vi "Test I8 Value.vi"(7 "Name":string="Test I8 Value", 8 "Upper Limit":refnum<class "Abs_I8 Integer.lvclass">, 9 "Lower Limit":refnum<class "Abs_I8 Integer.lvclass">, 10 "Limit Test Type":T1, 11 "Tested Value":refnum<class "Abs_I8 Integer.lvclass">) -> (3 "abs_Node":refnum<class "abs_Node.lvclass">)   [LabVIEW 2021, in "BT.lvlib"]
uses:
  BT.lvlib
  Support/Nodes/abs_Node/abs_Node.lvclass
  Support/Limit Test Type.ctl
  <vilib>/TSA/Abstract Data Classes/Abs_Types/I8 Integer/Abs_I8 Integer.lvclass
  C:/Program Files (x86)/National Instruments/LabVIEW 2021/vi.lib/TSA/Abstract Data Classes/Abs_Types/Numeric/Abs_Numeric.lvclass
  Support/Nodes/Leaves/Test Boolean/Test Boolean.lvclass
  C:/Program Files (x86)/National Instruments/LabVIEW 2021/vi.lib/TSA/Abstract Data Classes/Abs_Types/Type/Abs_Type.lvclass
  C:/Users/Tim/Documents/GitHub/LV_Behaviour_Tree/Source/Support/abs_Type Leaf/abs_Type Leaf.lvclass
  C:/Users/Tim/Documents/GitHub/LV_Behaviour_Tree/Source/Support/abs_Node/abs_Node.lvclass
  <vilib>/TSA/Abstract Data Classes/Abs_Types/Type/Abs_Type.lvclass/Abs_Type.ctl
  Support/Nodes/Leaves/abs_Type Leaf/abs_Type Leaf.lvclass/abs_Type Leaf.ctl
  <vilib>/TSA/Abstract Data Classes/Abs_Types/Type/Properties/Write Name.vi
  Support/Nodes/Leaves/abs_Type Leaf/Properties/Write Value Class.vi
  <vilib>/TSA/Abstract Data Classes/Abs_Types/Boolean/Abs_Boolean.lvclass
  <vilib>/TSA/Abstract Data Classes/Functions/Compare/Support/Equal/I8/Method.vi
  <vilib>/TSA/Abstract Data Classes/Functions/Compare/Support/Not Equal/I8/Method.vi
  <vilib>/TSA/Abstract Data Classes/Functions/Compare/Support/Greater/I8/Method.vi
  <vilib>/TSA/Abstract Data Classes/Functions/Compare/Support/Less/I8/Method.vi
  <vilib>/TSA/Abstract Data Classes/Functions/Compare/Support/Greater Equal/I8/Method.vi
  <vilib>/TSA/Abstract Data Classes/Functions/Compare/Support/Less Equal/I8/Method.vi
  <vilib>/TSA/Abstract Data Classes/Functions/Logic/Support/AND/Bool/Method.vi
  <vilib>/TSA/Abstract Data Classes/Functions/Logic/Support/OR/Bool/Method.vi
  <vilib>/TSA/Abstract Data Classes/Functions/Math/Support/Add/I8/Method.vi
  <vilib>/TSA/Abstract Data Classes/Functions/Math/Support/Subtract/I8/Method.vi
  <vilib>/TSA/Abstract Data Classes/Functions/Logic/Support/AND/Bool/AND_Bool.lvclass
  <vilib>/TSA/Abstract Data Classes/Functions/Logic/Support/OR/Bool/OR_Bool.lvclass
  <vilib>/TSA/Abstract Data Classes/Functions/Compare/Support/Equal/I8/Equal_I8.lvclass
  <vilib>/TSA/Abstract Data Classes/Functions/Compare/Support/Not Equal/I8/Not Equal_I8.lvclass
  <vilib>/TSA/Abstract Data Classes/Functions/Compare/Support/Greater/I8/Greater_I8.lvclass
  <vilib>/TSA/Abstract Data Classes/Functions/Compare/Support/Less/I8/Less_I8.lvclass
  <vilib>/TSA/Abstract Data Classes/Functions/Compare/Support/Greater Equal/I8/Greater Equal_I8.lvclass
  <vilib>/TSA/Abstract Data Classes/Functions/Compare/Support/Less Equal/I8/Less Equal_I8.lvclass
  C:/Program Files (x86)/National Instruments/LabVIEW 2021/vi.lib/TSA/Abstract Data Classes/Abs_Types/Integer/Abs_Integer.lvclass
  C:/Program Files (x86)/National Instruments/LabVIEW 2021/vi.lib/TSA/Abstract Data Classes/Abs_Types/Value/Abs_Value.lvclass
  C:/Program Files (x86)/National Instruments/LabVIEW 2021/vi.lib/TSA/Abstract Data Classes/Abs_Types/I8 Integer/Abs_I8 Integer.lvclass
  <vilib>/TSA/Abstract Data Classes/Functions/Math/Support/Add/I8/Add_I8.lvclass
  <vilib>/TSA/Abstract Data Classes/Functions/Math/Support/Subtract/I8/Subtract_I8.lvclass
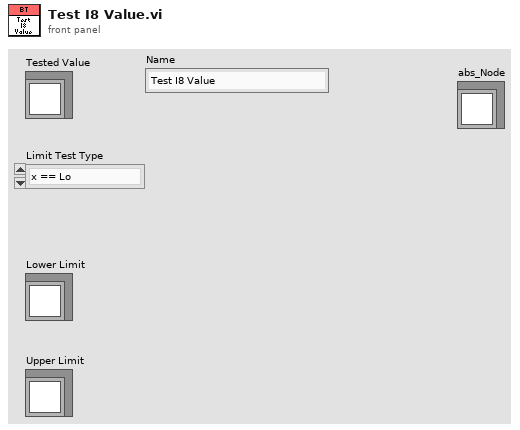
[diagram p1: front panel]
types:
  T1 = typedef "BT.lvlib/Limit Test Type.ctl" = enum16{"x == Lo", "x != Lo", "x > Lo", "x < Lo", "x >= Lo", "x <= Lo", "Lo > x < Hi", "Lo >= x <= Hi", "Lo >= x < Hi", "Lo > x <= Hi", "Lo < x > Hi", "Lo <= x >= Hi", "Lo <= x > Hi", "Lo < x >= Hi", "x == Lo +/- Hi"}
  T2 = typedef "Add_I8.lvclass/Abs_Type.ctl" = refnum<class "Abs_I8 Integer.lvclass">
  T3 = typedef "Subtract_I8.lvclass/Abs Type.ctl" = refnum<class "Abs_I8 Integer.lvclass">
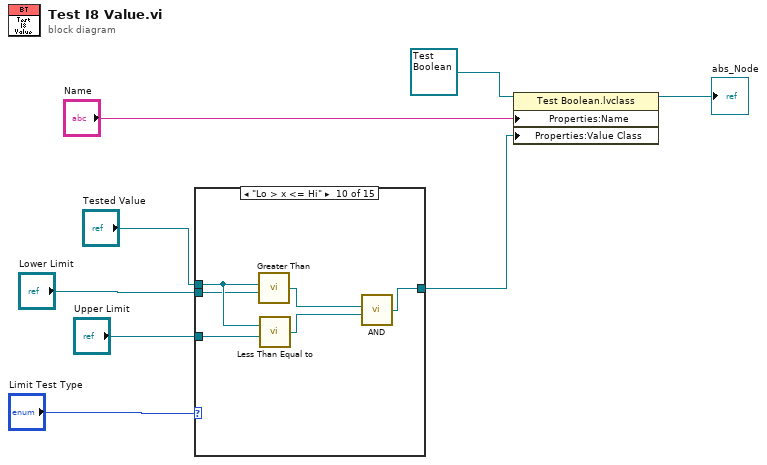
[diagram p0: block diagram]
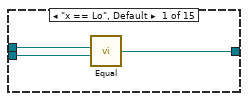
[diagram p2: hidden frame]
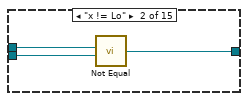
[diagram p3: hidden frame]
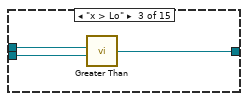
[diagram p4: hidden frame]
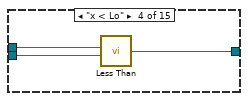
[diagram p5: hidden frame]
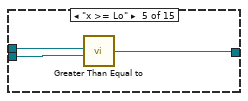
[diagram p6: hidden frame]
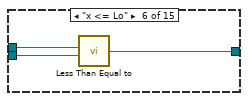
[diagram p7: hidden frame]
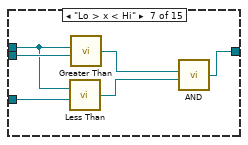
[diagram p8: hidden frame]
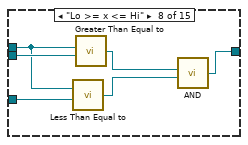
[diagram p9: hidden frame]
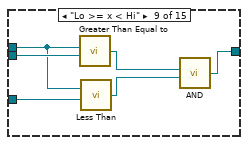
[diagram p10: hidden frame]
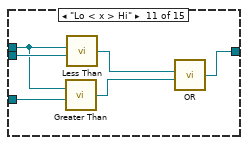
[diagram p11: hidden frame]
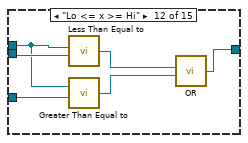
[diagram p12: hidden frame]
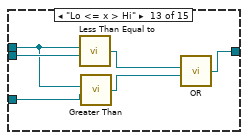
[diagram p13: hidden frame]
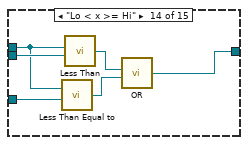
[diagram p14: hidden frame]
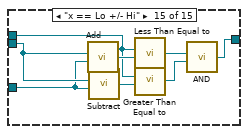
[diagram p15: hidden frame]
diagram:
  n1 = case shown="\"Lo > x <= Hi\"" "Limit Test Type" {
    tunnel: "Tested Value" -> [w11 w13 w17 w20 w23 w26 w31 w37 w43 w49 w53 w61 w66 w72 w79]
    tunnel: "Lower Limit" -> [w10 w14 w16 w19 w22 w25 w32 w38 w44 w48 w55 w62 w68 w73 w82]
    tunnel: [w9 w12 w15 w18 w21 w24 w27 w33 w39 w45 w56 w57 w63 w69 w75] -> w3
    tunnel: "Upper Limit" -> [_ _ _ _ _ _ w30 w36 w42 w50 w54 w60 w67 w74 w81]
    frame "x == Lo", Default {
      n2 = call-poly <vilib>:"Equal.vi"("Value B"=w10, "Value A"=w11) -> ("Result"=w9:refnum<class "Abs_Boolean.lvclass">)  [unwired: 4 in]
    }
    frame "x != Lo" {
      n3 = call-poly <vilib>:"Not Equal.vi"("Value B"=w14, "Value A"=w13) -> ("Result"=w12:refnum<class "Abs_Boolean.lvclass">)  [unwired: 4 in]
    }
    frame "x > Lo" {
      n4 = call-poly <vilib>:"Greater Than.vi"("Value B"=w16, "Value A"=w17) -> ("Result"=w15:refnum<class "Abs_Boolean.lvclass">)  [unwired: 4 in]
    }
    frame "x < Lo" {
      n5 = call-poly <vilib>:"Less Than.vi"("Value B"=w19, "Value A"=w20) -> ("Result"=w18:refnum<class "Abs_Boolean.lvclass">)  [unwired: 4 in]
    }
    frame "x >= Lo" {
      n6 = call-poly <vilib>:"Greater Than Equal to.vi"("Value B"=w22, "Value A"=w23) -> ("Result"=w21:refnum<class "Abs_Boolean.lvclass">)  [unwired: 4 in]
    }
    frame "x <= Lo" {
      n7 = call-poly <vilib>:"Less Than Equal to.vi"("Value B"=w25, "Value A"=w26) -> ("Result"=w24:refnum<class "Abs_Boolean.lvclass">)  [unwired: 4 in]
    }
    frame "Lo > x < Hi" {
      n8 = call-poly <vilib>:"Less Than.vi"("Value B"=w30, "Value A"=w31) -> ("Result"=w28:refnum<class "Abs_Boolean.lvclass">)  [unwired: 4 in]
      n9 = call-poly <vilib>:"Greater Than.vi"("Value B"=w32, "Value A"=w31) -> ("Result"=w29:refnum<class "Abs_Boolean.lvclass">)  [unwired: 4 in]
      n10 = call-poly <vilib>:"AND.vi"("B"=w28, "A"=w29) -> ("Result"=w27:refnum<class "Abs_Boolean.lvclass">)  [unwired: 4 in]
    }
    frame "Lo >= x <= Hi" {
      n11 = call-poly <vilib>:"Less Than Equal to.vi"("Value B"=w36, "Value A"=w37) -> ("Result"=w34:refnum<class "Abs_Boolean.lvclass">)  [unwired: 4 in]
      n12 = call-poly <vilib>:"Greater Than Equal to.vi"("Value B"=w38, "Value A"=w37) -> ("Result"=w35:refnum<class "Abs_Boolean.lvclass">)  [unwired: 4 in]
      n13 = call-poly <vilib>:"AND.vi"("B"=w34, "A"=w35) -> ("Result"=w33:refnum<class "Abs_Boolean.lvclass">)  [unwired: 4 in]
    }
    frame "Lo >= x < Hi" {
      n14 = call-poly <vilib>:"Greater Than Equal to.vi"("Value B"=w44, "Value A"=w43) -> ("Result"=w40:refnum<class "Abs_Boolean.lvclass">)  [unwired: 4 in]
      n15 = call-poly <vilib>:"Less Than.vi"("Value B"=w42, "Value A"=w43) -> ("Result"=w41:refnum<class "Abs_Boolean.lvclass">)  [unwired: 4 in]
      n16 = call-poly <vilib>:"AND.vi"("B"=w41, "A"=w40) -> ("Result"=w39:refnum<class "Abs_Boolean.lvclass">)  [unwired: 4 in]
    }
    frame "Lo > x <= Hi" {
      n17 = call-poly <vilib>:"Greater Than.vi"("Value B"=w48, "Value A"=w49) -> ("Result"=w47:refnum<class "Abs_Boolean.lvclass">)  [unwired: 4 in]
      n18 = call-poly <vilib>:"Less Than Equal to.vi"("Value B"=w50, "Value A"=w49) -> ("Result"=w46:refnum<class "Abs_Boolean.lvclass">)  [unwired: 4 in]
      n19 = call-poly <vilib>:"AND.vi"("B"=w46, "A"=w47) -> ("Result"=w45:refnum<class "Abs_Boolean.lvclass">)  [unwired: 4 in]
    }
    frame "Lo < x > Hi" {
      n20 = call-poly <vilib>:"Greater Than.vi"("Value B"=w54, "Value A"=w53) -> ("Result"=w51:refnum<class "Abs_Boolean.lvclass">)  [unwired: 4 in]
      n21 = call-poly <vilib>:"Less Than.vi"("Value B"=w55, "Value A"=w53) -> ("Result"=w52:refnum<class "Abs_Boolean.lvclass">)  [unwired: 4 in]
      n22 = call-poly <vilib>:"OR.vi"("B"=w51, "A"=w52) -> ("Result"=w56:refnum<class "Abs_Boolean.lvclass">)  [unwired: 4 in]
    }
    frame "Lo <= x >= Hi" {
      n23 = call-poly <vilib>:"Less Than Equal to.vi"("Value B"=w62, "Value A"=w61) -> ("Result"=w58:refnum<class "Abs_Boolean.lvclass">)  [unwired: 4 in]
      n24 = call-poly <vilib>:"Greater Than Equal to.vi"("Value B"=w60, "Value A"=w61) -> ("Result"=w59:refnum<class "Abs_Boolean.lvclass">)  [unwired: 4 in]
      n25 = call-poly <vilib>:"OR.vi"("B"=w59, "A"=w58) -> ("Result"=w57:refnum<class "Abs_Boolean.lvclass">)  [unwired: 4 in]
    }
    frame "Lo <= x > Hi" {
      n26 = call-poly <vilib>:"Less Than Equal to.vi"("Value B"=w68, "Value A"=w66) -> ("Result"=w65:refnum<class "Abs_Boolean.lvclass">)  [unwired: 4 in]
      n27 = call-poly <vilib>:"Greater Than.vi"("Value B"=w67, "Value A"=w66) -> ("Result"=w64:refnum<class "Abs_Boolean.lvclass">)  [unwired: 4 in]
      n28 = call-poly <vilib>:"OR.vi"("B"=w64, "A"=w65) -> ("Result"=w63:refnum<class "Abs_Boolean.lvclass">)  [unwired: 4 in]
    }
    frame "Lo < x >= Hi" {
      n29 = call-poly <vilib>:"Less Than Equal to.vi"("Value B"=w74, "Value A"=w72) -> ("Result"=w70:refnum<class "Abs_Boolean.lvclass">)  [unwired: 4 in]
      n30 = call-poly <vilib>:"Less Than.vi"("Value B"=w73, "Value A"=w72) -> ("Result"=w71:refnum<class "Abs_Boolean.lvclass">)  [unwired: 4 in]
      n31 = call-poly <vilib>:"OR.vi"("B"=w70, "A"=w71) -> ("Result"=w69:refnum<class "Abs_Boolean.lvclass">)  [unwired: 4 in]
    }
    frame "x == Lo +/- Hi" {
      n32 = call-poly <vilib>:"Add.vi"("Input B"=w81, "Input A"=w82) -> ("Result"=w80:T2)  [unwired: 4 in]
      n33 = call-poly <vilib>:"Subtract.vi"("Input B"=w81, "Input A"=w82) -> ("Result"=w78:T3)  [unwired: 4 in]
      n34 = call-poly <vilib>:"Less Than Equal to.vi"("Value B"=w80, "Value A"=w79) -> ("Result"=w77:refnum<class "Abs_Boolean.lvclass">)  [unwired: 4 in]
      n35 = call-poly <vilib>:"Greater Than Equal to.vi"("Value B"=w78, "Value A"=w79) -> ("Result"=w76:refnum<class "Abs_Boolean.lvclass">)  [unwired: 4 in]
      n36 = call-poly <vilib>:"AND.vi"("B"=w76, "A"=w77) -> ("Result"=w75:refnum<class "Abs_Boolean.lvclass">)  [unwired: 4 in]
    }
  }
  n37 = property class="Test Boolean.lvclass"(reference=refnum<class "Test Boolean.lvclass"> refnum ("BT.lvlib:Test Boolean.lvclass"), "Properties:Name"="Name", "Properties:Value Class"=w3) -> (reference out=→"abs_Node":refnum<class "Test Boolean.lvclass">)  [unwired: 1 in, 1 out]
